vi "Set - Append Signals to wForm.vi"(0 "reference in":refnum<class "GSwFormDSP.lvclass">, 5 "error in (no error)":errorcluster, 7 "New Signals":waveform(dbl)[](array[waveform])) -> (14 "reference out":refnum<class "GSwFormDSP.lvclass">, 19 "error out":errorcluster)   [LabVIEW 2022 SP3, in "GSwFormDSP.lvclass"]
uses:
  GSwFormDSP.lvclass
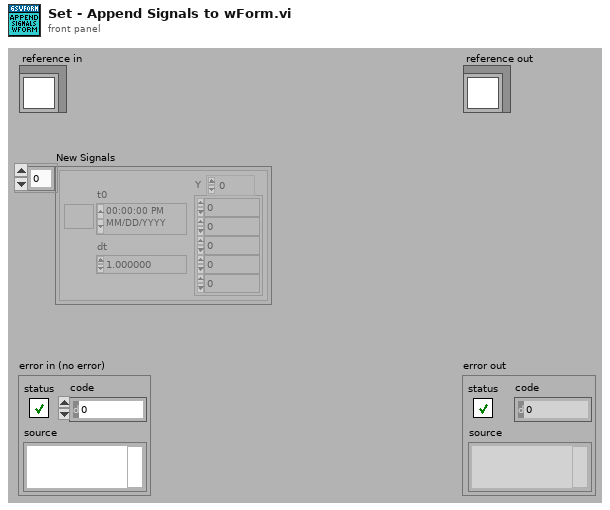
[diagram p1: front panel]
types:
  T1 = typedef "GSwFormDSP.lvclass/ObjectAttributesRef.ctl" = refnum<data-value>
  T2 = typedef "GSwFormDSP.lvclass/ObjectAttributes.ctl" = cluster{"Wform Ref":refnum<data-value>, "Nb Signals":i32, "Spectral Function Parameters":T3, "FFT":waveform(cdb)[], "Nb FFT":i32, "Nb Averages":i32[], "Reference Indexes":i32[], "Response Indexes":i32[], "Coherence":waveform(dbl)[], "TDF Parameters":T5, "DAQ":cluster{"Duration (sec)":dbl, "Buffer Size (Samples)":i32, "Offset (Samples)":i32}, "Filter Impulse Response (TDF)":waveform(dbl), "Sound Playback":T6}
  T3 = typedef "GSwFormDSP.lvclass/Spectral Parameters.ctl" = cluster{"Frequency resolution (Hz)":dbl, "Overlap":dbl, "Window":T4}
  T4 = typedef "NI_AALPro.lvlib/windowTd.ctl" = u32
  T5 = typedef "GSwFormDSP.lvclass/TDF Parameters.ctl" = cluster{"Filter":enum32{"Lowpass", "Highpass", "Bandpass", "Bandstop"}, "Type:":enum16{"Butterworth", "Chebyshev", "Inv Chebyshev", "Elliptic", "Bessel"}, "LP cutoff freq":dbl, "HP cutoff freq":dbl, "Order":i32, "passband ripple (dB)":dbl, "stopband attenuation (dB)":dbl, "Phaseless Filter":bool, "Include Fade IN and OUT":bool}
  T6 = typedef "GSwFormDSP.lvclass/Sound Playback.ctl" = cluster{"Timer start (ms)":u32, "task ID":T7, "Cursor Init Location (s)":dbl, "SC Volume":dbl}
  T7 = typedef "Sound Output Task ID.ctl" = u32
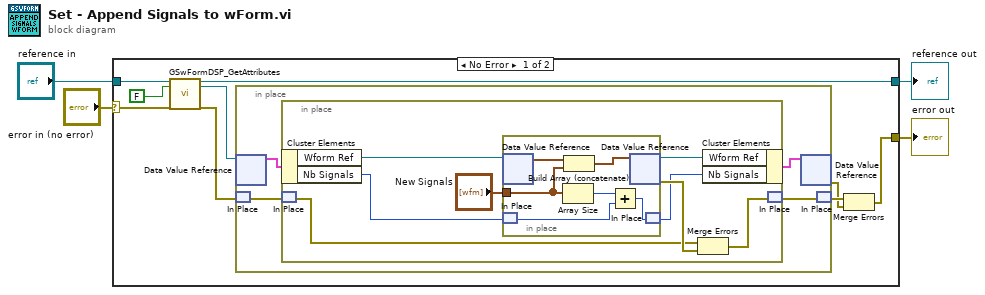
[diagram p0: block diagram]
diagram:
  n1 = case shown="No Error" "error in (no error)" {
    selector: "error in (no error)" -> [w11 w33]
    tunnel: [w5 w33] -> w3
    tunnel: [w6 w32] -> w1
    tunnel: "reference in" -> [w13 w32]
    frame No Error {
      n2 = call "GSwFormDSP_GetAttributes.vi"("reference in"=w13, "return data? (T)"=FALSE, "error in (no error)"=w11) -> ("reference out"=w6:refnum<class "GSwFormDSP.lvclass">, "attributes ref"=w10:T1, "error out"=w9:errorcluster)  [unwired: 13 in, 1 out]
      n3 = in-place {
        n4 = in-place-dvr #1(w10) -> (w16:T2)  [unwired: 1 out]
        n5 = in-place-match #2(w9) -> (w15:errorcluster)
        n6 = in-place {
          n7 = in-place-cluster #3(w16) -> ("Wform Ref"=w25:refnum<data-value>, "Nb Signals"=w19:i32)
          n8 = in-place-match #4(w15) -> (w21:errorcluster)
          n9 = in-place {
            in-place-border: "New Signals" -> [w29]
            n10 = in-place-dvr #5(w25) -> (w31:waveform(dbl)[])  [unwired: 1 out]
            n11 = in-place-match #6(w19) -> (w27:i32)
            n12 = Array Size(array=w29) -> (size(s)=w28:i32)
            n13 = Build Array (concatenate)(w31, w29) -> (w30:waveform(dbl)[])
            n14 = Add(x=w28, y=w27) -> (x+y=w26:i32)
            n15 = in-place-dvr #5(w30) -> (w24:refnum<data-value>, w22:errorcluster)
            n16 = in-place-match #6(w26) -> (w18:i32)
          }
          n17 = Merge Errors(w21, w22) -> (w20:errorcluster)
          n18 = in-place-cluster #3("Wform Ref"=w24, "Nb Signals"=w18) -> (w17:T2)
          n19 = in-place-match #4(w20) -> (w14:errorcluster)
        }
        n20 = in-place-dvr #1(w17) -> (w7:errorcluster)  [unwired: 1 out]
        n21 = in-place-match #2(w14) -> (w8:errorcluster)
      }
      n22 = Merge Errors(w8, w7) -> (w5:errorcluster)
    }
    frame Error {
    }
  }
  "error out" <- w3
  "reference out" <- w1
